vi "Read RootPath.vi"(8 "error in (no error)":errorcluster, 11 "WebBrowser_Mgmt in":refnum<class "WebBrowser_Mgmt.lvclass">) -> (0 "error out":errorcluster, 2 "RootPath":path, 3 "WebBrowser_Mgmt out":refnum<class "WebBrowser_Mgmt.lvclass">)   [LabVIEW 2016, in "WebBrowser_Mgmt.lvclass"]
uses:
  WebBrowser_Mgmt.lvclass
  WebBrowser_Mgmt.lvclass/WebBrowser_Mgmt.ctl
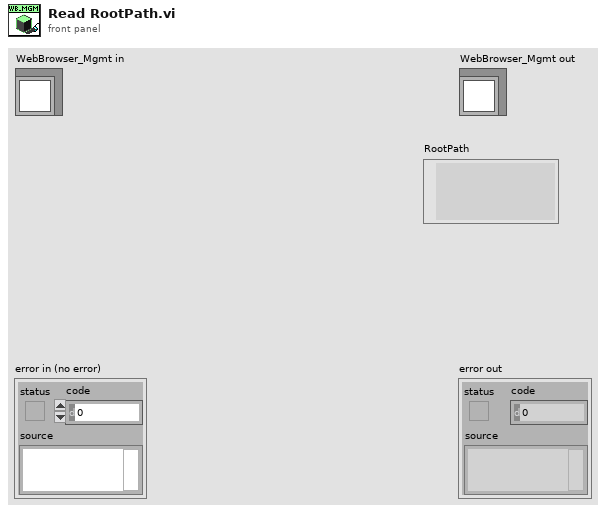
[diagram p1: front panel]
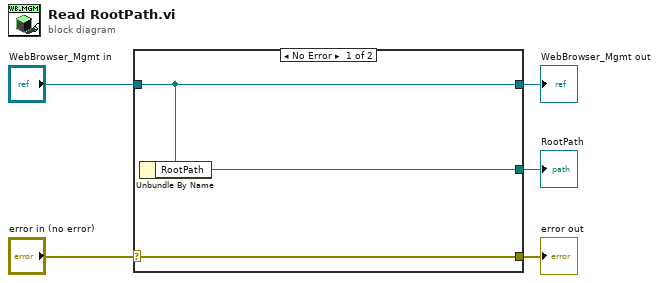
[diagram p0: block diagram]
diagram:
  n1 = case shown="No Error" "error in (no error)" {
    selector: "error in (no error)" -> [w8 w9]
    tunnel: [w8 w9] -> w4
    tunnel: [w7 w10] -> w2
    tunnel: "WebBrowser_Mgmt in" -> [w7 w10]
    tunnel: [w6 _] -> w1
    frame No Error {
      n2 = Unbundle By Name(w7) -> ("RootPath"=w6:path)
    }
    frame Error {
    }
  }
  "error out" <- w4
  "WebBrowser_Mgmt out" <- w2
  "RootPath" <- w1
